vi "Configure Channel.vi"(0 "VISA resource name":refnum<visa-resource-name>, 1 "Enable Channel (Enable)":bool=TRUE, 2 "BW Limit 20MHz (Disable)":bool, 3 "Input Impedance (1: 1 Mohms)":u32(ring)=1 items=["50 ohms", "1 Mohms"], 5 "Channel (1: Channel 1)":i32(ring)=1 items=["Channel 1"=1, "Channel 2"=2, "Channel 3"=3, "Channel 4"=4], 7 "Vertical Coupling (1: DC)":i32(ring)=1 items=["AC", "DC"], 9 "Probe Attenuation (1.0)":dbl=1.0, 11 "error in (no error)":errorcluster, 12 "Vertical Range (2.0 V)":dbl=2.0, 13 "Vertical Offset (0.0 V)":dbl) -> (4 "VISA resource name out":refnum<visa-resource-name>, 15 "error out":errorcluster)   [LabVIEW 2012, in "Agilent 8000 Series.lvlib"]
doc: "Configures the common properties of the vertical subsystem of the oscilloscope for the specified channel. Call this VI for each channel you want to enable to acquire waveforms.\n\n<B>Note:</B>\nThe channel settings will not be applied if the channel is not enabled."
uses:
  Agilent 8000 Series.lvlib
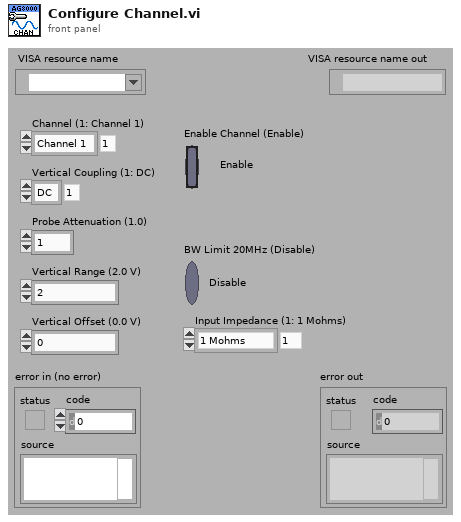
[diagram p1: front panel]
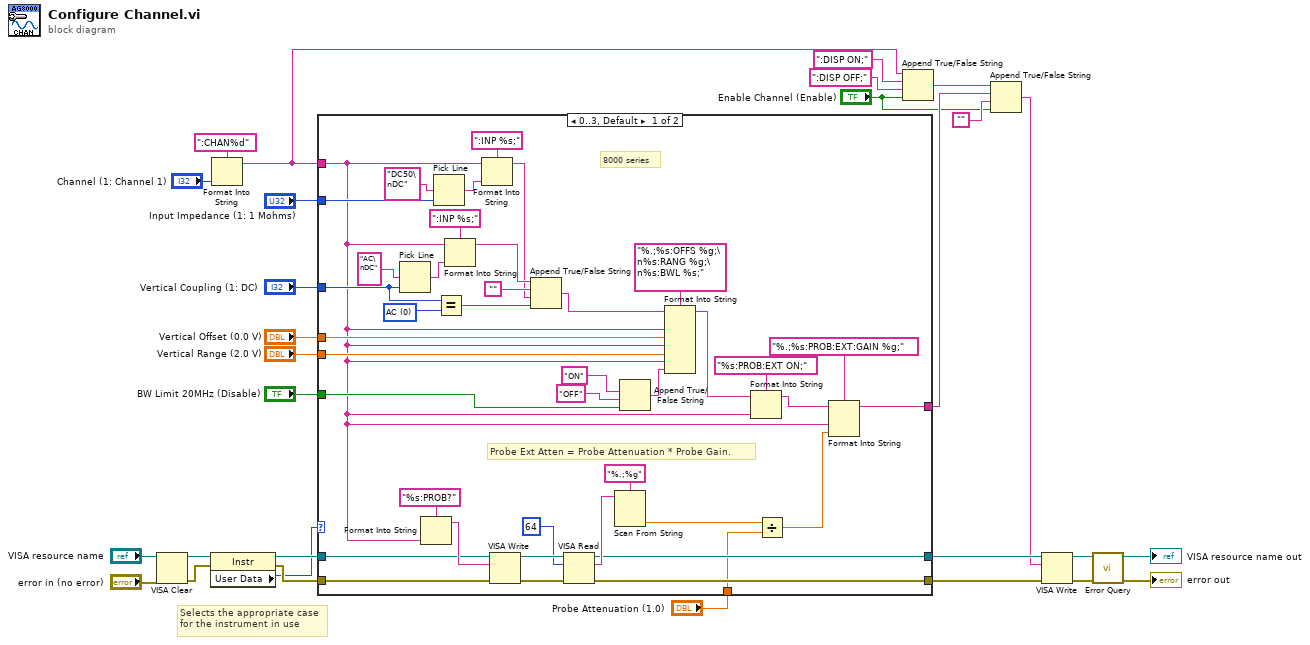
[diagram p0: block diagram]
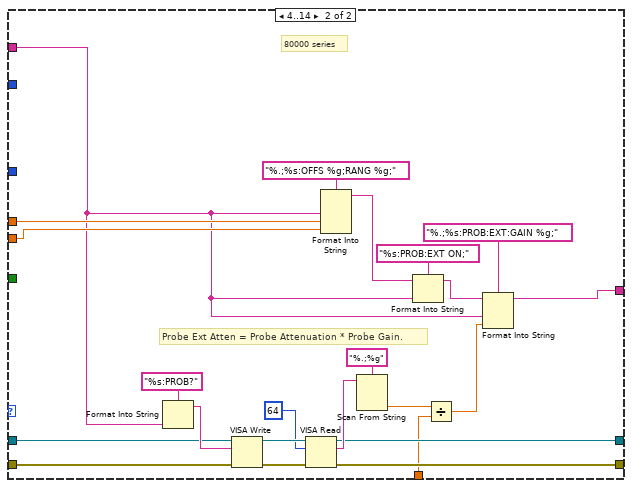
[diagram p2: hidden frame]
diagram:
  # "Selects the appropriate case\nfor the instrument in use"
  n1 = VISA Clear(VISA resource name="VISA resource name", error in (no error)="error in (no error)") -> (VISA resource name out=w2:refnum<visa-resource-name>, error out=w1:errorcluster)
  n2 = property class="Instr"(reference=w2, error in=w1) -> (reference out=w21:refnum<visa-resource-name>, error out=w20:errorcluster, "User Data"=w19:u32)
  n3 = Format Into String(format string=":CHAN%d", "Channel (1: Channel 1)") -> (resulting string=w5:string)  [unwired: 2 in, 1 out]
  n4 = case shown="0..3, Default" w19 {
    tunnel: w5 -> [w30 w71]
    tunnel: w21 -> [w67 w90]
    tunnel: w20 -> [w66 w89]
    tunnel: [w58 w81] -> w23
    tunnel: [w40 w77] -> w22
    tunnel: [w39 w76] -> w9
    tunnel: "Input Impedance (1: 1 Mohms)" -> [w37 _]
    tunnel: "Vertical Coupling (1: DC)" -> [w36 _]
    tunnel: "Vertical Offset (0.0 V)" -> [w35 w74]
    tunnel: "Vertical Range (2.0 V)" -> [w32 w73]
    tunnel: "Probe Attenuation (1.0)" -> [w34 w72]
    tunnel: "BW Limit 20MHz (Disable)" -> [w33 _]
    frame 0..3, Default {
      w49 = 0 items=["AC", "DC"]
      # "8000 series"
      # "Probe Ext Atten = Probe Attenuation * Probe Gain."
      n5 = Pick Line(multi-line string="AC\nDC", line index=w36) -> (output string=w50:string)  [unwired: 1 in]
      n6 = Format Into String(format string="%s:PROB?", w30) -> (resulting string=w68:string)  [unwired: 2 in, 1 out]
      n7 = Pick Line(multi-line string="DC50\nDC", line index=w37) -> (output string=w53:string)  [unwired: 1 in]
      n8 = Equal?(x=w36, y=w49) -> (x = y?=w48:bool)
      n9 = Format Into String(format string=":INP %s;", initial string=w30, w50) -> (resulting string=w47:string)  [unwired: 1 in, 1 out]
      n10 = Format Into String(format string=":INP %s;", initial string=w30, w53) -> (resulting string=w45:string)  [unwired: 1 in, 1 out]
      n11 = VISA Write(VISA resource name=w67, write buffer=w68, error in (no error)=w66) -> (VISA resource name out=w65:refnum<visa-resource-name>, error out=w64:errorcluster)  [unwired: 1 out]
      n12 = Append True/False String(1:w48, 2:w45, 3:"", 4:w47) -> (0:w44:string)
      n13 = VISA Read(VISA resource name=w65, byte count=u32 64, error in (no error)=w64) -> (VISA resource name out=w58:refnum<visa-resource-name>, read buffer=w62:string, error out=w40:errorcluster)  [unwired: 1 out]
      n14 = Scan From String(format string="%.;%g", input string=w62) -> (output 1=w59:dbl)  [unwired: 3 in, 3 out]
      n15 = Append True/False String(1:w33, 2:"OFF" ("true string"), 3:"ON" ("true string")) -> (0:w31:string)  [unwired: 1 in]
      n16 = Format Into String(format string="%.;%s:OFFS %g;\n%s:RANG %g;\n%s:BWL %s;", initial string=w44, w30, w35, w30, w32, w30, w31) -> (resulting string=w43:string)  [unwired: 1 in, 1 out]
      n17 = Format Into String(format string="%s:PROB:EXT ON;", initial string=w43, w30) -> (resulting string=w38:string)  [unwired: 1 in, 1 out]
      n18 = Divide(x=w59, y=w34) -> (x/y=w60:dbl)
      n19 = Format Into String(format string="%.;%s:PROB:EXT:GAIN %g;", initial string=w38, w30, w60) -> (resulting string=w39:string)  [unwired: 1 in, 1 out]
    }
    frame 4..14 {
      # "80000 series"
      # "Probe Ext Atten = Probe Attenuation * Probe Gain."
      n20 = Format Into String(format string="%s:PROB?", w71) -> (resulting string=w91:string)  [unwired: 2 in, 1 out]
      n21 = VISA Write(VISA resource name=w90, write buffer=w91, error in (no error)=w89) -> (VISA resource name out=w88:refnum<visa-resource-name>, error out=w87:errorcluster)  [unwired: 1 out]
      n22 = VISA Read(VISA resource name=w88, byte count=u32 64, error in (no error)=w87) -> (VISA resource name out=w81:refnum<visa-resource-name>, read buffer=w85:string, error out=w77:errorcluster)  [unwired: 1 out]
      n23 = Format Into String(format string="%.;%s:OFFS %g;RANG %g;", w71, w74, w73) -> (resulting string=w79:string)  [unwired: 2 in, 1 out]
      n24 = Scan From String(format string="%.;%g", input string=w85) -> (output 1=w82:dbl)  [unwired: 3 in, 3 out]
      n25 = Format Into String(format string="%s:PROB:EXT ON;", initial string=w79, w71) -> (resulting string=w75:string)  [unwired: 1 in, 1 out]
      n26 = Divide(x=w82, y=w72) -> (x/y=w83:dbl)
      n27 = Format Into String(format string="%.;%s:PROB:EXT:GAIN %g;", initial string=w75, w71, w83) -> (resulting string=w76:string)  [unwired: 1 in, 1 out]
    }
  }
  n28 = Append True/False String(1:"Enable Channel (Enable)", 2:":DISP OFF;" ("false string"), 3:":DISP ON;" ("true string"), 4:w5) -> (0:w10:string)
  n29 = Append True/False String(1:"Enable Channel (Enable)", 2:"", 3:w9, 4:w10) -> (0:w6:string)
  n30 = VISA Write(VISA resource name=w23, write buffer=w6, error in (no error)=w22) -> (VISA resource name out=w27:refnum<visa-resource-name>, error out=w26:errorcluster)  [unwired: 1 out]
  n31 = call "Error Query.vi"("error in (no error)"=w26, "VISA resource name"=w27) -> ("error out"=→"error out":errorcluster, "VISA resource name out"=→"VISA resource name out":refnum<visa-resource-name>)  [unwired: 6 in, 2 out]
